vi "Time.vi"() -> (0 "Time":string, 1 "Date":string, 2 "Formatted time":string)   [LabVIEW 2021]
uses:
  <vilib>/regexp/Match Regular Expression.xnode
panel:
  out "PM_AM":string
  out "Minute":string
  out "Hour":string
  out "Year":string
  out "Day":string
  out "Month":string
  out "time string":string
  out "date string":string
  out "current time":timestamp
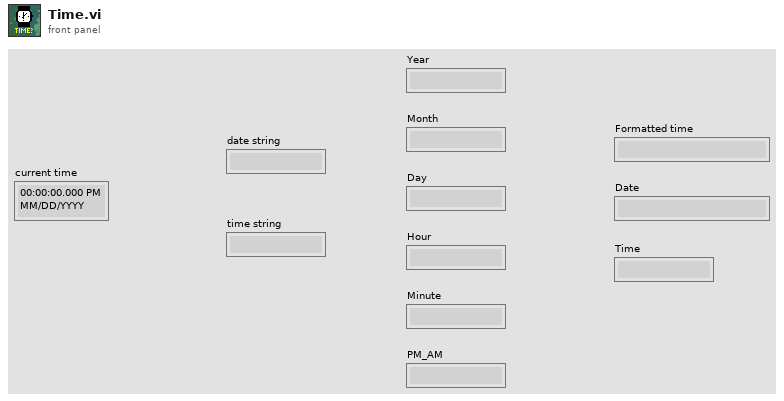
[diagram p1: front panel]
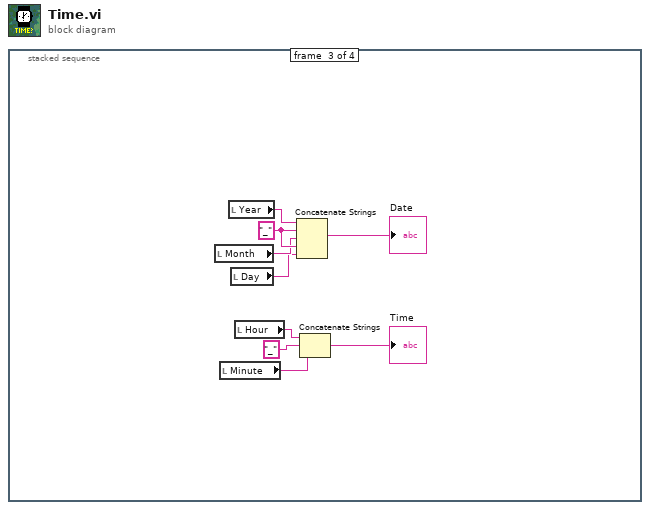
[diagram p0: block diagram]
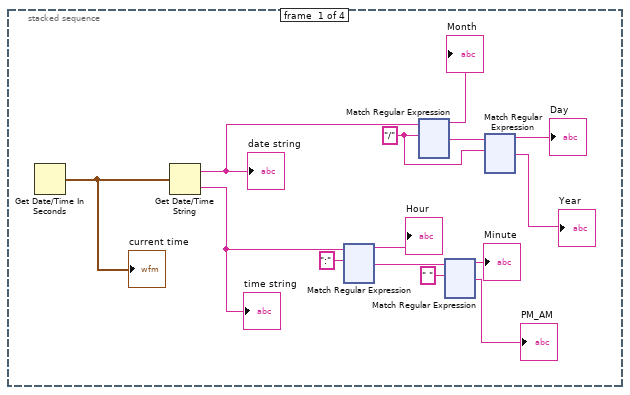
[diagram p2: hidden frame]
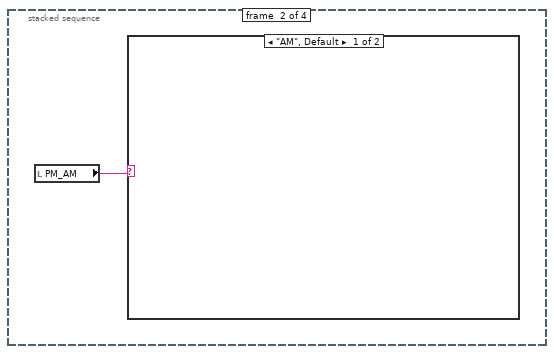
[diagram p3: hidden frame]
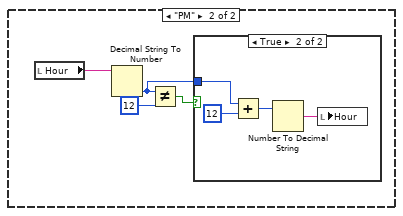
[diagram p4: hidden frame]
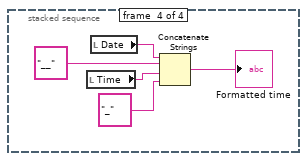
[diagram p6: hidden frame]
diagram:
  n1 = stacked-sequence {
    frame #0 {
      w11 = "/" ("regular expression")
      n2 = Get Date/Time In Seconds() -> (seconds since 1Jan1904=w14:timestamp)
      "current time" <- w14
      n3 = Get Date/Time String(seconds (now)=w14) -> (date string=w13:string, time string=w7:string)  [unwired: 2 in]
      "date string" <- w13
      "time string" <- w7
      n4 = xnode "Match Regular Expression"("input string"=w7, "regular expression"=":") -> ("before match"=→"Hour":string, "after match"=w6:string)  [unwired: 4 in, 3 out]
      n5 = xnode "Match Regular Expression"("input string"=w13, "regular expression"=w11) -> ("before match"=→"Month":string, "after match"=w12:string)  [unwired: 4 in, 3 out]
      n6 = xnode "Match Regular Expression"("input string"=w6, "regular expression"=" ") -> ("before match"=→"Minute":string, "after match"=→"PM_AM":string)  [unwired: 4 in, 3 out]
      n7 = xnode "Match Regular Expression"("input string"=w12, "regular expression"=w11) -> ("before match"=→"Day":string, "after match"=→"Year":string)  [unwired: 4 in, 3 out]
    }
    frame #1 {
      n8 = local read "PM_AM"() -> (w483:string)
      n9 = case shown="\"AM\", Default" w483 {
        frame "AM", Default {
        }
        frame "PM" {
          n10 = local read "Hour"() -> (w487:string)
          n11 = Decimal String To Number(string=w487) -> (number=w485:i32)  [unwired: 2 in, 1 out]
          n12 = Not Equal?(x=w485, y=12) -> (x != y?=w484:bool)
          n13 = case shown="True" w484 {
            tunnel: w485 -> [_ w488]
            frame False {
            }
            frame True {
              n14 = Add(x=w488, y=12) -> (x+y=w490:i32)
              n15 = Number To Decimal String(number=w490) -> (decimal integer string=w489:string)  [unwired: 1 in]
              n16 = local write "Hour"(w489) -> ()
            }
          }
        }
      }
    }
    frame #2 {
      w499 = "_" ("string")
      n17 = local read "Month"() -> (w497:string)
      n18 = local read "Minute"() -> (w494:string)
      n19 = local read "Year"() -> (w498:string)
      n20 = local read "Day"() -> (w496:string)
      n21 = local read "Hour"() -> (w495:string)
      n22 = Concatenate Strings(w498, w499, w497, w499, w496) -> (→"Date":string)
      n23 = Concatenate Strings(w495, "_" ("string"), w494) -> (→"Time":string)
    }
    frame #3 {
      n24 = local read "Time"() -> (w503:string)
      n25 = local read "Date"() -> (w504:string)
      n26 = Concatenate Strings(w504, "__" ("string"), w503, "_" ("string")) -> (→"Formatted time":string)
    }
  }
